vi "sCMOS_get_last_image.vi"(1 "Image In":T1, 2 "Frame Index":i32=-1, 3 "Error in":errorcluster, 4 "Handle in":u32) -> (6 "image error":errorcluster={"status"=FALSE, "code"=0, "source"="Simple acquisition.vi->GetMostRecentImage.vi"})   [LabVIEW 2015]
uses:
  <vilib>/vision/Image Controls.llb/IMAQ Image.ctl
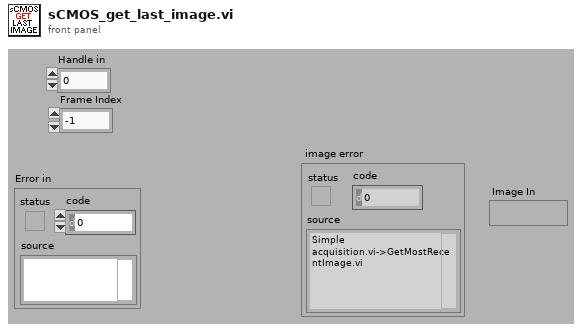
[diagram p1: front panel]
types:
  T1 = typedef "IMAQ Image.ctl" = refnum<image>
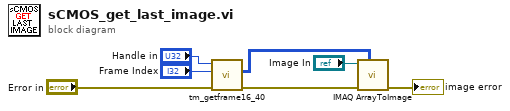
[diagram p0: block diagram]
diagram:
  n1 = call <userlib>:"tm_getframe16_40.vi"("error in (no error)"="Error in", "Frame Index"="Frame Index", "Handle in"="Handle in") -> ("error out"=w3:errorcluster, "Data"=w1:u16[][])  [unwired: 5 in, 2 out]
  n2 = call "IMAQ ArrayToImage"("Image Pixels (U16)"=w1, "error in (no error)"=w3, "Image"="Image In") -> ("error out"=→"image error":errorcluster)  [unwired: 7 in, 1 out]
